vi "novoGoleiro.vi"(9 "balls":T1[](array[typedef]), 10 "Robot in":T3, 11 "IA State":T2={"our_robots"=[], "enemy_robots"=[], "balls"=[], "geometry"={"field_length"=0, "field_width"=0, "goal_width"=0, "goal_depth"=0, "center_circle_radius"=0, "defense_width"=0, "defense_depth"=0, "free_kick_from_defense_dist"=0, "penalty_spot_from_field_line_dist"=0, "penalty_line_from_spot_dist"=0, "half_moon_depth"=0, "half_moon_width"=0}, "IA Judge"={"stage"="", "command"="", "our_goalie_id"=0.0, "enemy_goalie_id"=0.0, "command enum"=enum."Halt", "Time"=enum."Azul"}, "Received Timestamp"=timestamp(0 s since 1904-01-01), "Events"={"Touch"=FALSE, "id touch"=0.0, "Ball out of \nVision"=FALSE, "Ball inside \nGoalie area"=FALSE, "Robot not responding"=FALSE, "Robots responding status"=[1.0, 1.0, 1.0, 1.0, 1.0, 1.0], "Enemy Ball \nPossession"=FALSE, "Id ini Possession"=0.0, "Ball Possesion"=FALSE, "Id Possesion"=0.0, "Ball at\nour goal side"=FALSE, "Ball at\ntouchline"=FALSE, "Ball at\nenemy goal side"=FALSE}}) -> (3 "Robot out":T3)   [LabVIEW 2018]
uses:
  Core/AI Robot.ctl
  Intel/Functions Enum.ctl
  Intel/AttackerStates.ctl
  Path Planning/RRT/PathDests.ctl
  Path Planning/RRT/PathDest.ctl
  Core/AI Input.ctl
  Core/AI Ball.ctl
  Core/Field Size.ctl
  Core/AI Judge.ctl
  Intel/Command Enum.ctl
  Util/Events/Events.ctl
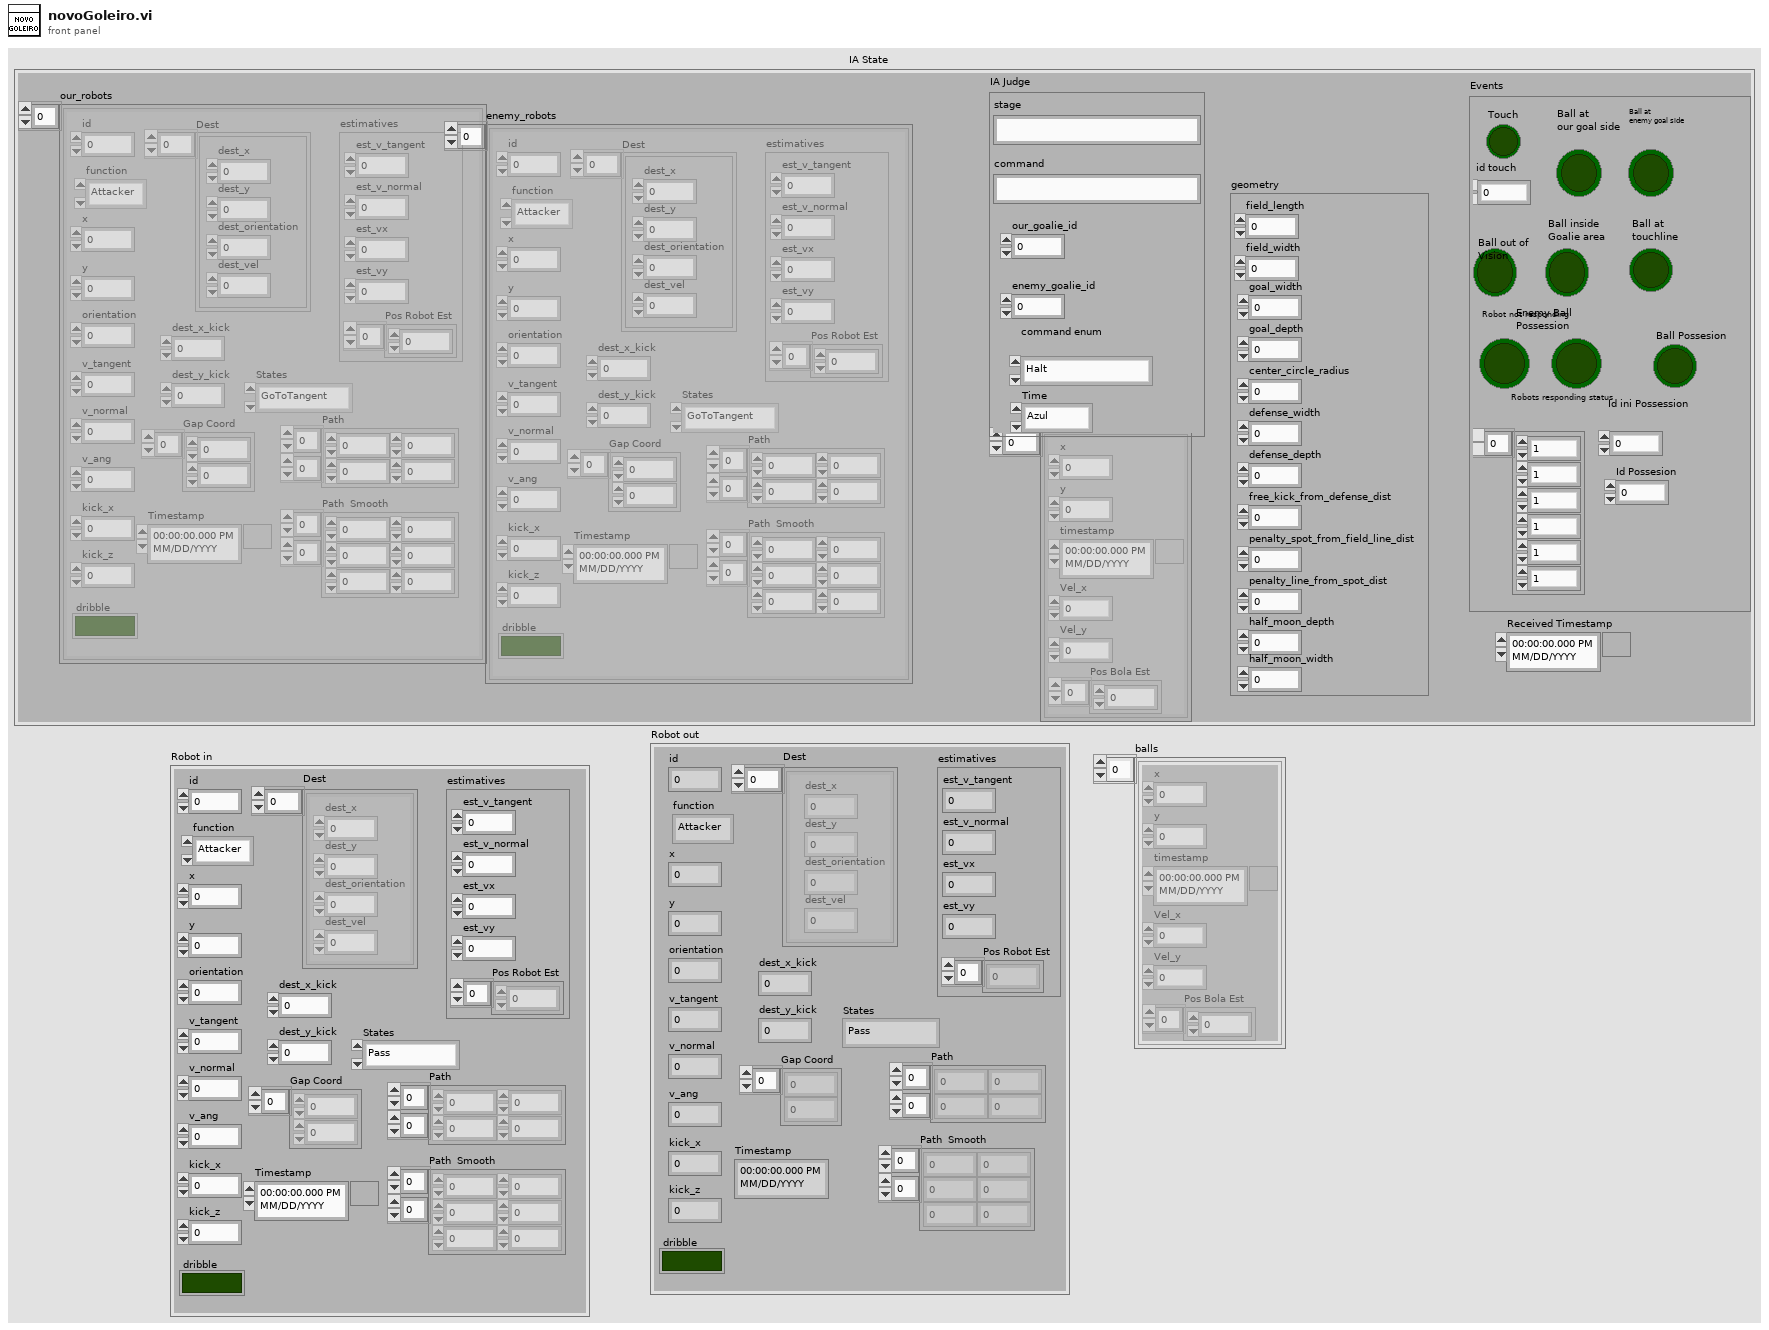
[diagram p1: front panel]
types:
  T1 = typedef "AI Ball.ctl" = cluster{"x":dbl, "y":dbl, "timestamp":timestamp, "Vel_x":dbl, "Vel_y":dbl, "Pos Bola Est":dbl[]}
  T2 = typedef "AI Input.ctl" = cluster{"our_robots":T3[], "enemy_robots":T3[], "balls":T1[], "geometry":T8, "IA Judge":T9, "Received Timestamp":timestamp, "Events":T11}
  T3 = typedef "AI Robot.ctl" = cluster{"id":u32, "function":T4, "x":dbl, "y":dbl, "orientation":dbl, "v_tangent":dbl, "v_normal":dbl, "v_ang":dbl, "kick_x":dbl, "kick_z":dbl, "dribble":bool, "Timestamp":timestamp, "estimatives":cluster{"est_v_tangent":dbl, "est_v_normal":dbl, "est_vx":dbl, "est_vy":dbl, "Pos Robot Est":dbl[]}, "dest_x_kick":dbl, "dest_y_kick":dbl, "Gap Coord":dbl[], "States":T5, "Path ":dbl[][], "Path  Smooth":dbl[][], "Dest":T6}
  T4 = typedef "Functions Enum.ctl" = enum16{"Attacker", "Goalie", "Defender", "Striker", "Goto 0", "Dummy", "Kicker", "ZigZag"}
  T5 = typedef "AttackerStates.ctl" = enum16{"Pass", "GoToTangent", "BallGetting", "GoToKick", "Rotate anti-clockwise", "Rotate Clockwise", ""}
  T6 = typedef "PathDests.ctl" = T7[]
  T7 = typedef "PathDest.ctl" = cluster{"dest_x":dbl, "dest_y":dbl, "dest_orientation":dbl, "dest_vel":dbl}
  T8 = typedef "Field Size.ctl" = cluster{"field_length":u32, "field_width":u32, "goal_width":u32, "goal_depth":u32, "center_circle_radius":u32, "defense_width":u32, "defense_depth":u32, "free_kick_from_defense_dist":u32, "penalty_spot_from_field_line_dist":u32, "penalty_line_from_spot_dist":u32, "half_moon_depth":u32, "half_moon_width":u32}
  T9 = typedef "AI Judge.ctl" = cluster{"stage":string, "command":string, "our_goalie_id":dbl, "enemy_goalie_id":dbl, "command enum":T10, "Time":enum16{"Azul", "Amarelo"}}
  T10 = typedef "Command Enum.ctl" = enum16{"Halt", "Stop", "Force Start", "PKA Normal Start", "Prepare Kickoff Ally", "PKE Normal Start", "Prepare Kickoff Enemy", "Prepare Penalty Ally", "PPA Normal Start", "Prepare Penalty Enemy", "PPE Normal Start", "Ball Placement Enemy Up", "Ball Placement Enemy Down", "Ball Placement Ally Up", "Ball Placement Ally Mid", "Ball Placement Ally Down", "Indirect Free Enemy", "Indirect Free Ally", "Timeout Enemy", "Timeout Ally", "Goal Enemy", "Goal Ally", "Normal Half Time", "Extra Time Break", "Extra Half Time", "None", "Post Game"}
  T11 = typedef "Events.ctl" = cluster{"Touch":bool, "id touch":dbl, "Ball out of \nVision":bool, "Ball inside \nGoalie area":bool, "Robot not responding":bool, "Robots responding status":dbl[], "Enemy Ball \nPossession":bool, "Id ini Possession":dbl, "Ball Possesion":bool, "Id Possesion":dbl, "Ball at\nour goal side":bool, "Ball at\ntouchline":bool, "Ball at\nenemy goal side":bool}
  T12 = enum16{"Goleiro fora da área", "Alinhar com a bola", "Alinhar com a trave", "Rotacionar", "Aproximar-se da bola", "Posicionar-se na frente da bola"}
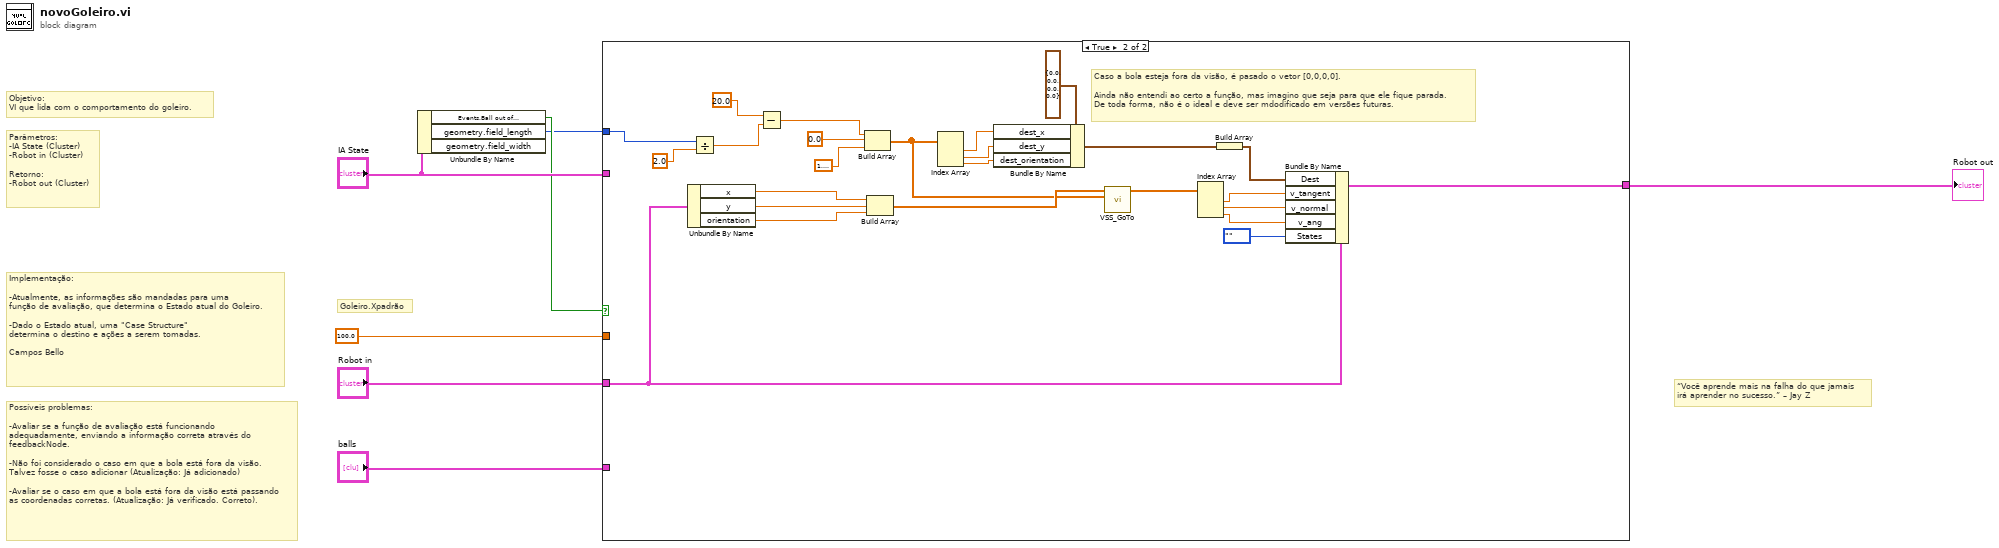
[diagram p0: block diagram]
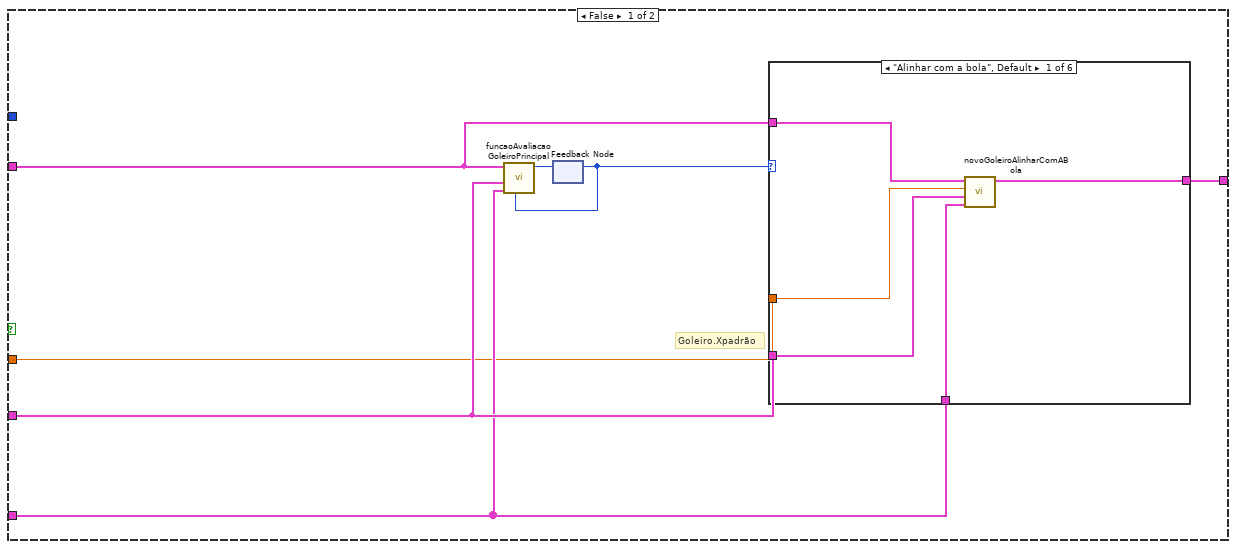
[diagram p2: hidden frame]
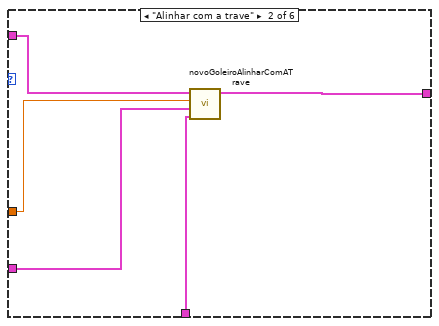
[diagram p3: hidden frame]
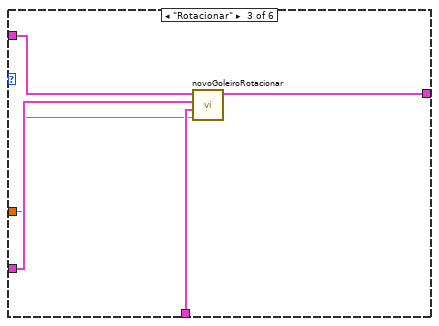
[diagram p4: hidden frame]
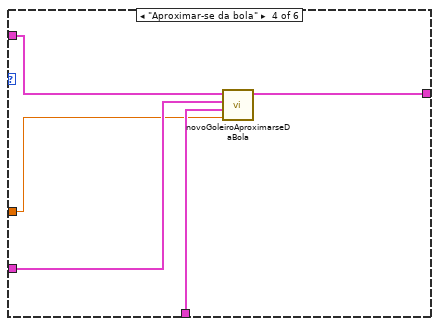
[diagram p5: hidden frame]
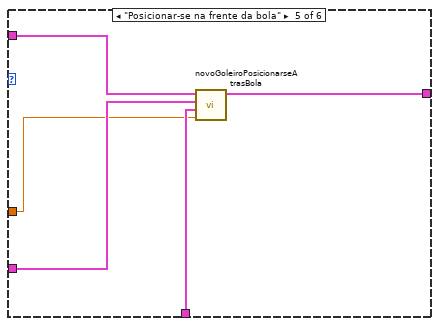
[diagram p6: hidden frame]
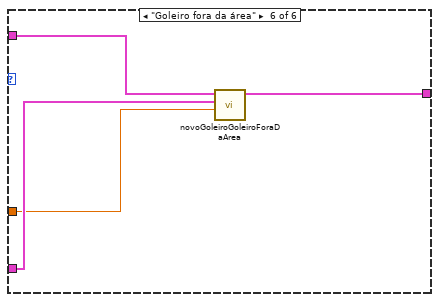
[diagram p7: hidden frame]
diagram:
  # "“Você aprende mais na falha do que jamais \nirá aprender no sucesso.” – Jay Z"
  # "Possíveis problemas:\n\n-Avaliar se a função de avaliação está funcionando\nadequadamente, enviando a informação correta através do\nfeedbackNode.\n\n-Não foi considerado o caso em que a bola está fora da visão.\nTalvez fosse o caso adicionar (Atualização: Já adicionado)\n\n-Avaliar se o caso em que a bola está fora da visão está passando\nas coordenadas corretas. (Atualização: Já verificado. Correto)."
  # "Implementação:\n\n-Atualmente, as informações são mandadas para uma \nfunção de avaliação, que determina o Estado atual do Goleiro.\n\n-Dado o Estado atual, uma \"Case Structure\" \ndetermina o destino e ações a serem tomadas.\n\nCampos Bello"
  # "Parâmetros:\n-IA State (Cluster)\n-Robot in (Cluster)\n\nRetorno:\n-Robot out (Cluster)"
  # "Objetivo:\nVI que lida com o comportamento do goleiro."
  # "Goleiro.Xpadrão"
  n1 = Unbundle By Name("IA State") -> ("Events.Ball out of \nVision"=w3:bool, "geometry.field_length"=w1:u32)  [unwired: 1 out]
  n2 = case shown="True" w3 {
    tunnel: 100.0 -> [w8 _]
    tunnel: "Robot in" -> [w12 w62]
    tunnel: [w14 w67] -> w5
    tunnel: "IA State" -> [w13 _]
    tunnel: "balls" -> [w11 _]
    tunnel: w1 -> [_ w49]
    frame False {
      # "Goleiro.Xpadrão"
      n3 = feedback #1() -> (w9:T12)  [unwired: 1 in]
      n4 = call "funcaoAvaliacaoGoleiroPrincipal.vi"("Estado_Goleiro Atual"=w9, "balls"=w11, "Robot in"=w12, "IA State"=w13) -> ("Estado_Goleiro"=w10:T12)  [unwired: 7 in]
      n5 = feedback-in #1(w10) -> ()
      n6 = case shown="\"Alinhar com a bola\", Default" w9 {
        tunnel: w13 -> [w19 w24 w29 w34 w39 w43]
        tunnel: [w17 w22 w28 w33 w37 w40] -> w14
        tunnel: w8 -> [w18 w23 w25 w30 w35 w41]
        tunnel: w12 -> [w16 w21 w27 w32 w38 w42]
        tunnel: w11 -> [w15 w20 w26 w31 w36 _]
        frame "Alinhar com a bola", Default {
          n7 = call "novoGoleiroAlinharComABola.vi"("balls"=w15, "Robot in"=w16, "Goleiro.X_padrao"=w18, "IA State"=w19) -> ("Cluster de saída"=w17:T3)  [unwired: 7 in]
        }
        frame "Alinhar com a trave" {
          n8 = call "novoGoleiroAlinharComATrave.vi"("balls"=w20, "Robot in"=w21, "Goleiro.X_padrao"=w23, "IA State"=w24) -> ("Cluster de saída"=w22:T3)  [unwired: 7 in]
        }
        frame "Rotacionar" {
          n9 = call "novoGoleiroRotacionar.vi"("Goleiro.X_padrao"=w25, "balls"=w26, "Robot in"=w27, "IA State"=w29) -> ("Cluster de saída"=w28:T3)  [unwired: 7 in]
        }
        frame "Aproximar-se da bola" {
          n10 = call "novoGoleiroAproximarseDaBola.vi"("Goleiro.X_padrao"=w30, "balls"=w31, "Robot in"=w32, "IA State"=w34) -> ("Cluster de saída"=w33:T3)  [unwired: 7 in]
        }
        frame "Posicionar-se na frente da bola" {
          n11 = call "novoGoleiroPosicionarseAtrasBola.vi"("Goleiro.X_padrao"=w35, "balls"=w36, "Robot in"=w38, "IA State"=w39) -> ("Cluster de saída"=w37:T3)  [unwired: 7 in]
        }
        frame "Goleiro fora da área" {
          n12 = call "novoGoleiroGoleiroForaDaArea.vi"("Goleiro.Xpadrão"=w41, "Robot in"=w42, "IA State"=w43) -> ("Cluster de saída"=w40:T3)  [unwired: 8 in]
        }
      }
    }
    frame True {
      # "Caso a bola esteja fora da visão, é pasado o vetor [0,0,0,0]. \n\nAinda não entendi ao certo a função, mas imagino que seja para que ele fique parada.\nDe toda forma, não é o ideal e deve ser mdodificado em versões futuras."
      n13 = Unbundle By Name(w62) -> ("x"=w61:dbl, "y"=w60:dbl, "orientation"=w59:dbl)
      n14 = Divide(x=w49, y=2.0) -> (x/y=w46:dbl)
      n15 = Subtract(x=20.0, y=w46) -> (x-y=w45:dbl)
      n16 = Build Array(w45, 0.0, 1.5707963267948966) -> (w54:dbl[])
      n17 = Build Array(w61, w60, w59) -> (w58:dbl[])
      n18 = Index Array(array=w54) -> (element #1=w53:dbl, element #2=w52:dbl, element #3=w51:dbl)  [unwired: 3 in]
      n19 = Bundle By Name(cluster=T7 {"dest_x"=0.0, "dest_y"=0.0, "dest_orientation"=0.0, "dest_vel"=0.0} ("element"), "dest_x"=w53, "dest_y"=w52, "dest_orientation"=w51) -> (w56:T7)
      n20 = call "VSS_GoTo.vi"("SetPoint"=w54, "Position"=w58) -> ("Output Vel"=w66:dbl[])  [unwired: 9 in]
      n21 = Index Array(array=w66) -> (element #1=w65:dbl, element #2=w64:dbl, element #3=w63:dbl)  [unwired: 3 in]
      n22 = Build Array(w56) -> (w55:T7[])
      n23 = Bundle By Name(cluster=w62, "Dest"=w55, "v_tangent"=w65, "v_normal"=w64, "v_ang"=w63, "States"=AttackerStates."") -> (w67:T3)
    }
  }
  "Robot out" <- w5
